vi "Calculate Thermistor Temp.vi"(11 "Numeric":dbl) -> (3 "Numeric 2":dbl)   [LabVIEW 2015]
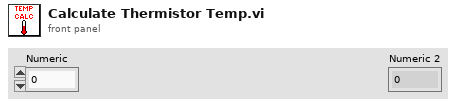
[diagram p1: front panel]
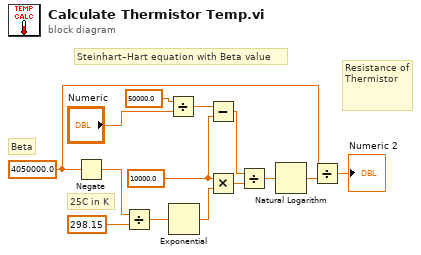
[diagram p0: block diagram]
diagram:
  w1 = 4050000.0
  w9 = 10000.0
  # "Steinhart–Hart equation with Beta value"
  # "25C in K"
  # "Resistance of\nThermistor"
  # "Beta"
  n1 = Negate(x=w1) -> (-x=w8:dbl)
  n2 = Divide(x=w8, y=298.15) -> (x/y=w6:dbl)
  n3 = Divide(x=50000.0, y="Numeric") -> (x/y=w12:dbl)
  n4 = Exponential(1:w6) -> (0:w5:dbl)
  n5 = Subtract(x=w12, y=w9) -> (x-y=w10:dbl)
  n6 = Multiply(x=w9, y=w5) -> (x*y=w4:dbl)
  n7 = Divide(x=w10, y=w4) -> (x/y=w3:dbl)
  n8 = Natural Logarithm(1:w3) -> (0:w11:dbl)
  n9 = Divide(x=w1, y=w11) -> (x/y=→"Numeric 2":dbl)
